vi "external enqueue command.vi"(8 "error in":errorcluster, 9 "Data":variant, 10 "Command":string, 11 "Queuename":string) -> (0 "error out":errorcluster, 3 "Queuename dup":string)   [LabVIEW 2013]
doc: "# #############################################################################\n# ATTENTION\n# #############################################################################\n#\n# This software is for guidance only. It is provided \"as is\".\n# It only aims at providing coding information to the customer in order for\n# them to save time. As a result no warranties, whether express, implied or\n# statutory, including, but not limited to implied warranties of\n# merchantability and fitness for a particular purpose apply to this software.\n# A·P·E Angewandte Physik und Elektronik GmbH shall not be held liable for any\n# direct, indirect or consequential damages with respect to any claims arising\n# from the content of such sourcecode and/or the use made by customers of the\n# coding information contained herein in connection with their products.\n#\n# #############################################################################"
uses:
  queue cluster.ctl
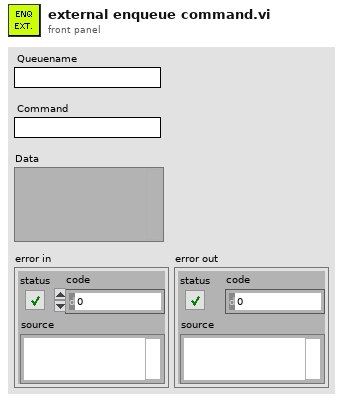
[diagram p1: front panel]
types:
  T1 = typedef "queue cluster.ctl" = cluster{"command":string, "data":variant}
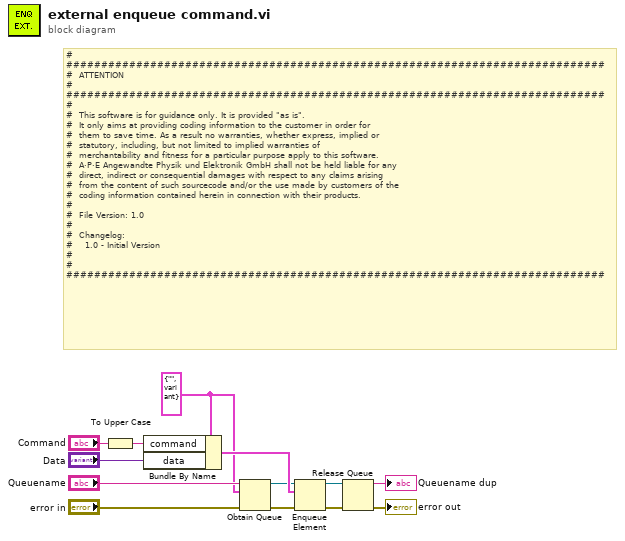
[diagram p0: block diagram]
diagram:
  w5 = T1 {"command"="", "data"=variant} ("QDSM Element")
  # "# #############################################################################\n#  ATTENTION\n# #############################################################################\n#\n#  This software is for guidance only. It is provided \"as is\".\n#  It only aims at providing coding information to the customer in order for\n#  them to save time. As a result no warranties, whether express, implied or\n#  statutory, including, but not limited to implied warranties of\n#  merchantability and fitness for a particular purpose apply to this software.\n#  A·P·E Angewandte Physik und Elektronik GmbH shall not be held liable for any\n#  direct, indirect or consequential damages with respect to any claims arising\n#  from the content of such sourcecode and/or the use made by customers of the\n#  coding information contained herein in connection with their products.\n#\n#  File Version: 1.0\n#\n#  Changelog:\n#    1.0 - Initial Version\n#\n# #############################################################################"
  n1 = To Upper Case(1:"Command") -> (0:w10:string)
  n2 = Bundle By Name(cluster=w5, "command"=w10, "data"="Data") -> (w13:T1)
  n3 = Obtain Queue(name (unnamed)="Queuename", element data type=w5, error in (no error)="error in") -> (queue out=w7:refnum<queue>, error out=w8:errorcluster)  [unwired: 2 in, 1 out]
  n4 = Enqueue Element(queue=w7, element=w13, error in (no error)=w8) -> (queue out=w2:refnum<queue>, error out=w4:errorcluster)  [unwired: 1 in, 1 out]
  n5 = Release Queue(queue=w2, error in (no error)=w4) -> (queue name=→"Queuename dup":string, error out=→"error out":errorcluster)  [unwired: 1 in, 1 out]
